vi "Connect to ACCDB Database.vi"() -> ()   [LabVIEW 2013]
doc: "This example demonstrates how to read data from a Microsoft Access 2007 database file. You must use the ACE engine instead of the JET engine to access the database. The example database file, Access2007.accdb, is located in the labview\\examples\\database directory.\n\nRun this VI to display all the data from the example ACCDB database. Examine the block diagram of this VI to see how to use the Database Variant To Data function to convert a database variant to the data type you need."
uses:
  Connection.llb/DB Tools Open Connec (String).vi
  _DB Variant To Data/Database Variant To Data.xnode
  NI_Database_API_64.lvlib
panel:
  out "error out":errorcluster
  out "Data returned from accdb file":cluster{string, i32, dbl}[](array[cluster])
  # "INSTRUCTIONS:\nThis example demonstrates how to read data from a Microsoft Access 2007 database file. You must use the ACE engine instead of the JET engine to access the database. The example database file, Access2007.accdb, is located in the labview\\examples\\database directory.\n\nRun this VI to display all the data from the example ACCDB database. Examine the block diagram of this VI to see how to use the Database Variant To Data function to convert a database variant to the data type you need.\n\nThis example VI requires the 2007 Office System Driver: Data Connectivity Components installed on the computer. You can download the components from the Microsoft Web site."
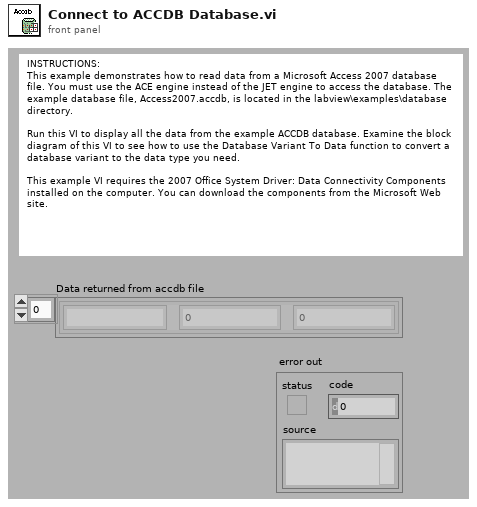
[diagram p1: front panel]
types:
  T1 = typedef "NI_Database_API_64.lvlib/Conn ObjectReference.ctl" = refnum<k1>
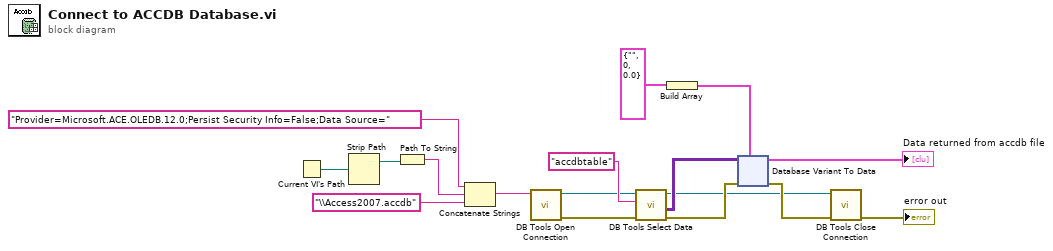
[diagram p0: block diagram]
diagram:
  n1 = Current VI's Path() -> (path=w6:path)
  n2 = Strip Path(path=w6) -> (stripped path=w4:path)  [unwired: 1 out]
  n3 = Path To String(path=w4) -> (string=w3:string)
  n4 = Concatenate Strings("Provider=Microsoft.ACE.OLEDB.12.0;Persist Security Info=False;Data Source=", w3, "\\Access2007.accdb") -> (w1:string)
  n5 = call-poly "DB Tools Open Connection.vi"("connection information"=w1) -> ("error out"=w15:errorcluster, "connection reference"=w16:T1)  [unwired: 7 in]
  n6 = call "DB Tools Select Data.vi"("error in (no error)"=w15, "table"="accdbtable" ("Table"), "connection reference"=w16) -> ("error out"=w10:errorcluster, "data"=w8:variant[][], "connection reference out"=w7:T1)  [unwired: 3 in]
  n7 = Build Array(cluster{string, i32, dbl} {"", 0, 0.0}) -> (w13:cluster{string, i32, dbl}[])
  n8 = xnode "Database Variant To Data"("database variant"=w8, "error in"=w10, "type"=w13) -> ("data"=→"Data returned from accdb file":cluster{string, i32, dbl}[], "error out"=w9:errorcluster)
  n9 = call "DB Tools Close Connection.vi"("error in (no error)"=w9, "connection reference"=w7) -> ("error out"=→"error out":errorcluster)  [unwired: 5 in]
